vi "Get Angle.vi"(6 "Axis":T1, 8 "error in (no error)":errorcluster, 11 "Instrument.Cryostat in":refnum<class "Instrument.Cryostat.lvclass">) -> (0 "error out":errorcluster, 1 "Status":string, 2 "Angle (°)":dbl, 3 "Instrument.Cryostat out":refnum<class "Instrument.Cryostat.lvclass">)   [LabVIEW 2019, in "Instrument.Cryostat.lvclass"]
uses:
  Instrument.Cryostat.lvclass
  Typedefs/Rotator Axis--Enum.ctl
panel:
  out "Finished?":bool
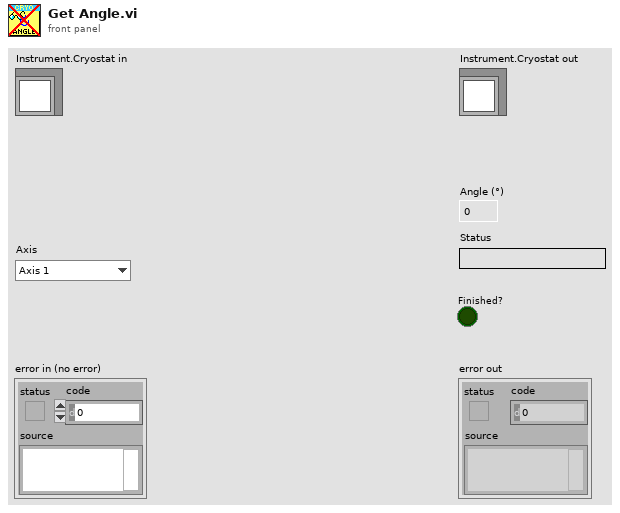
[diagram p1: front panel]
types:
  T1 = typedef "Instrument.Cryostat.lvclass/Rotator Axis--Enum.ctl" = enum16{"Axis 1", "Axis 2"}
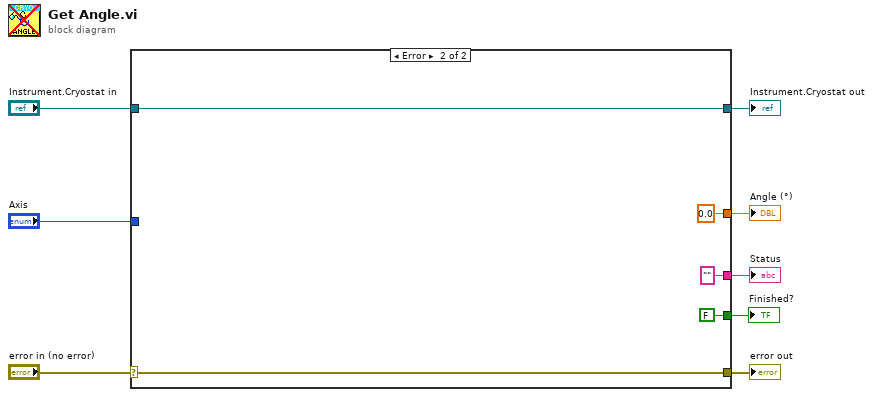
[diagram p0: block diagram]
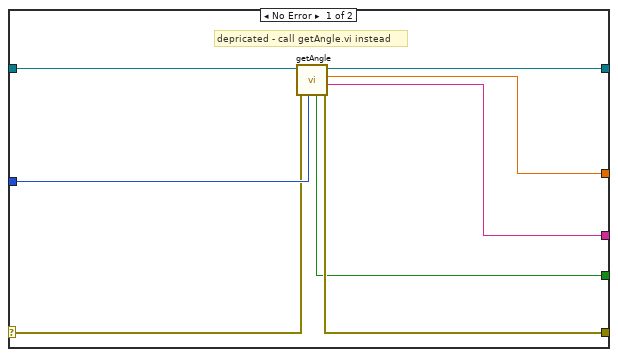
[diagram p2: hidden frame]
diagram:
  n1 = case shown="Error" "error in (no error)" {
    selector: "error in (no error)" -> [w13 w21]
    tunnel: [w12 w21] -> w7
    tunnel: [w16 w20] -> w5
    tunnel: "Instrument.Cryostat in" -> [w15 w20]
    tunnel: "Axis" -> [w14 _]
    tunnel: [w11 0.0 ("Angle (°)")] -> w3
    tunnel: [w10 "" ("Status")] -> w2
    tunnel: [w9 FALSE ("Finished?")] -> w1
    frame No Error {
      # "depricated - call getAngle.vi instead"
      n2 = call-dynamic "getAngle.vi"("Channel"=w14, "error in (no error)"=w13, "Instrument.Cryostat in"=w15) -> ("error out"=w12:errorcluster, "Status"=w10:string, "Angle (°)"=w11:dbl, "Instrument.Cryostat out"=w16:refnum<class "Instrument.Cryostat.lvclass">, "Finished?"=w9:bool)  [unwired: 4 in]
    }
    frame Error {
    }
  }
  "error out" <- w7
  "Instrument.Cryostat out" <- w5
  "Angle (°)" <- w3
  "Status" <- w2
  "Finished?" <- w1
